vi "Setup.vi"(8 "error in (no error)":errorcluster, 11 "UI View Test In":refnum<class "View Test.lvclass">) -> (0 "error out":errorcluster, 3 "UI View Test Out":refnum<class "View Test.lvclass">)   [LabVIEW 2020, in "View Test.lvclass"]
uses:
  View Test.lvclass
  C:/Git/astemes-triarc-framework/source/Framework Test/Base Class Test/Base Test.lvclass
  Framework/View/View.lvclass
  C:/Git/astemes-triarc-framework/source/Framework/Base/Base.lvclass
  Base Class Test/Base Test.lvclass/Base Test.ctl
  View Test.lvclass/View Test.ctl
  Base Class Test/Base Test.lvclass
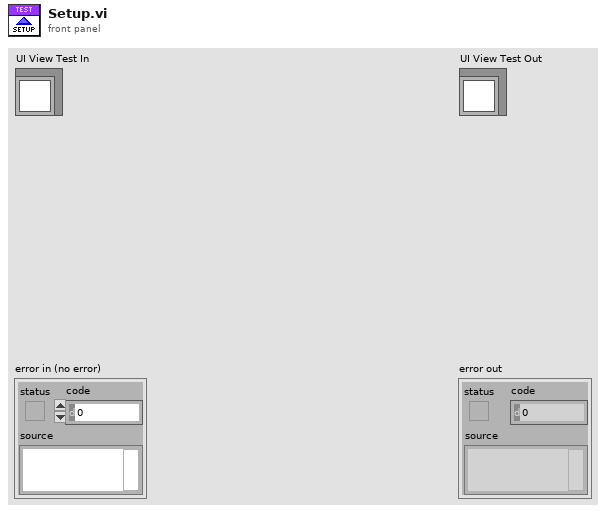
[diagram p1: front panel]
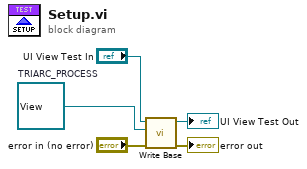
[diagram p0: block diagram]
diagram:
  w1 = refnum<class "View.lvclass"> refnum  # TRIARC_PROCESS
  n1 = call "Write Base.vi"("error in (no error)"="error in (no error)", "Base"=w1, "Base Class Test In"="UI View Test In") -> ("error out"=→"error out":errorcluster, "Base Class Test Out"=→"UI View Test Out":refnum<class "View Test.lvclass">)  [unwired: 7 in]
